vi "Get Picture.vi"(8 "error in (no error)":errorcluster, 11 "Metal Case in":refnum<class "Metal Case.lvclass">) -> (0 "error out":errorcluster, 2 "Picture":picture, 3 "Metal Case out":refnum<class "Metal Case.lvclass">)   [LabVIEW 2020, in "Metal Case.lvclass"]
uses:
  Metal Case.lvclass
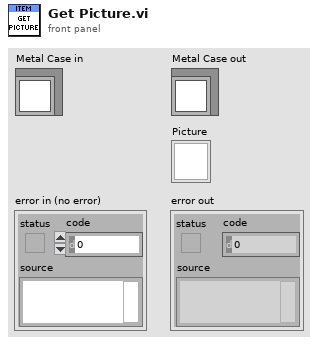
[diagram p1: front panel]
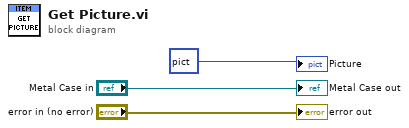
[diagram p0: block diagram]
diagram:
  "error out" <- "error in (no error)"
  "Metal Case out" <- "Metal Case in"
  "Picture" <- picture bytes[3230] ("new picture")
